vi "Programmatically Populate Tree Control_LV2012_NI Verified.vi"() -> ()   [LabVIEW 2015]
doc: "This VI shows how to programmatically populate a tree control using the Edit Tree Items.Add Item invoke node."
panel:
  in  "Tree":string(tree)
  # "Overview: This VI shows how to programmatically populate a tree control using the Edit Tree Items.Add Item invoke node.\nRequirements: LabVIEW 2012 (or compatible)\nInstructions:\nRun the VI"
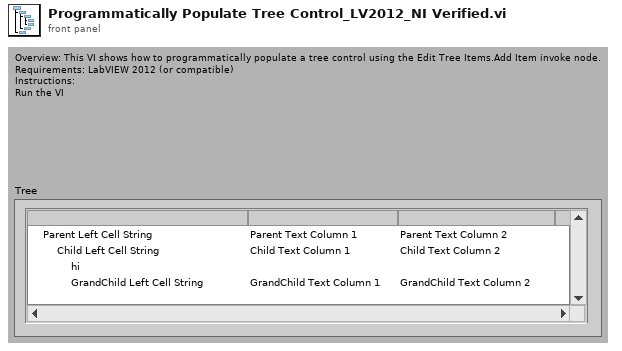
[diagram p1: front panel]
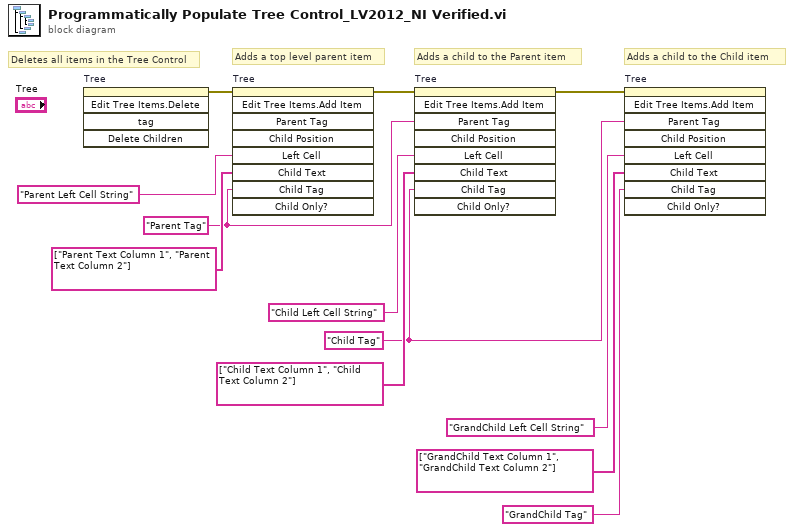
[diagram p0: block diagram]
diagram:
  w7 = "Parent Tag" ("Child Tag")
  w2 = "Child Tag" ("Child Tag")
  # "Adds a child to the Child item"
  # "Adds a child to the Parent item"
  # "Adds a top level parent item"
  # "Deletes all items in the Tree Control"
  n1 = invoke on="Tree" class="Tree (strict)" method="Edit Tree Items.Delete"() -> (error out=w9:errorcluster)  [unwired: 5 in, 4 out]
  n2 = invoke on="Tree" class="Tree (strict)" method="Edit Tree Items.Add Item"(error in=w9, "Left Cell"="Parent Left Cell String" ("Left Cell String"), "Child Text"=string[] ["Parent Text Column 1", "Parent Text Column 2"], "Child Tag"=w7) -> (error out=w12:errorcluster)  [unwired: 5 in, 8 out]
  n3 = invoke on="Tree" class="Tree (strict)" method="Edit Tree Items.Add Item"(error in=w12, "Parent Tag"=w7, "Left Cell"="Child Left Cell String" ("Left Cell String"), "Child Text"=string[] ["Child Text Column 1", "Child Text Column 2"], "Child Tag"=w2) -> (error out=w3:errorcluster)  [unwired: 4 in, 8 out]
  n4 = invoke on="Tree" class="Tree (strict)" method="Edit Tree Items.Add Item"(error in=w3, "Parent Tag"=w2, "Left Cell"="GrandChild Left Cell String" ("Left Cell String"), "Child Text"=string[] ["GrandChild Text Column 1", "GrandChild Text Column 2"], "Child Tag"="GrandChild Tag") -> ()  [unwired: 4 in, 9 out]
